vi "new_UI.vi"() -> ()   [LabVIEW 2019]
uses:
  Classes/Assembly/Assembly Run.lvclass
  Classes/Workspace/Fixture Enum.ctl
  Classes/Workspace/Fixture.lvclass
  Classes/Controller/Controller.lvclass
  Classes/Routine/Routine Enum.ctl
  Classes/Routine/Routine.lvclass
panel:
  in  "stop":bool
  in  "Add 2":bool
  in  "Go 2":bool
  in  "Cluster":T1
  in  "Remove":bool
  in  "Stage":i32(listbox)=-1
  in  "Add":bool
  in  "Routine":T2=enum."Dispense on Plate"
  in  "Update":bool
  out "Numeric":dbl
  out "Numeric 2":dbl
  in  "Stop":bool
  in  "Go":bool
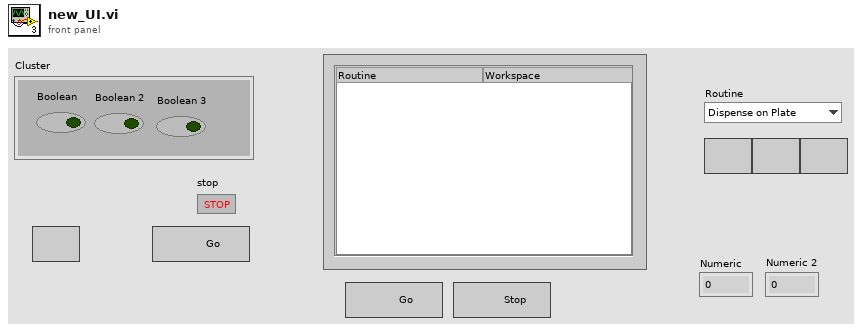
[diagram p1: front panel]
types:
  T1 = cluster{"Boolean":bool, "Boolean 2":bool, "Boolean 3":bool}
  T2 = typedef "Routine.lvclass/Routine Enum.ctl" = enum16{"Primary Pick Up", "Pick Up All", "Put Down Secondary", "Put Down All", "Release Syringe", "Secondary Pick Up", "Secure Syringe", "Dispense on Plate", "Dispense on Kapton", "Dispense on Sensor", "Dispense Offset"}
  T3 = typedef "Fixture.lvclass/Fixture Enum.ctl" = enum16{"Assembly Tray", "Syringe Space", "Component", "Pick Up Tool", "Current Position"}
  T4 = typedef "Controller.lvclass/Controllers.ctl" = cluster{"I-O.lvclass":refnum<class "I-O.lvclass">, "Dispenser.lvclass":refnum<class "Dispenser.lvclass">, "Gantry":refnum<k24>}
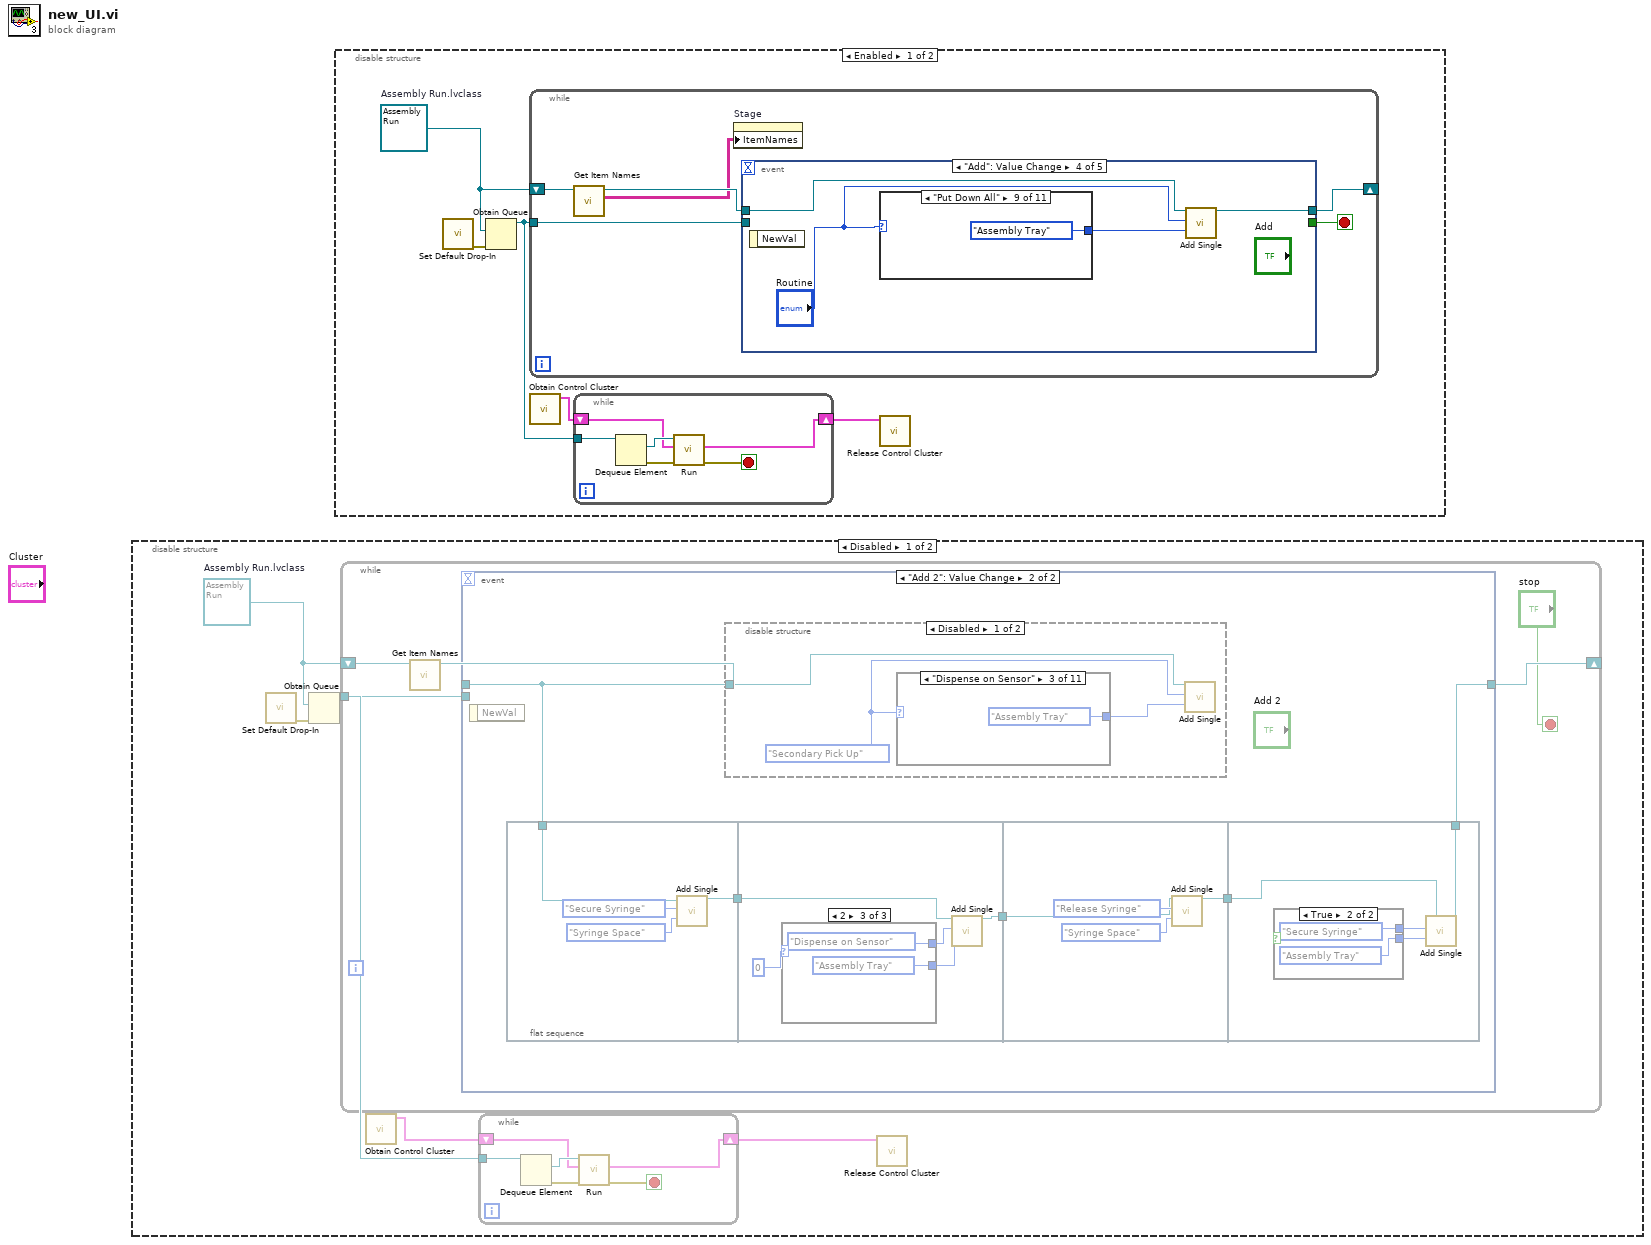
[diagram p0: block diagram]
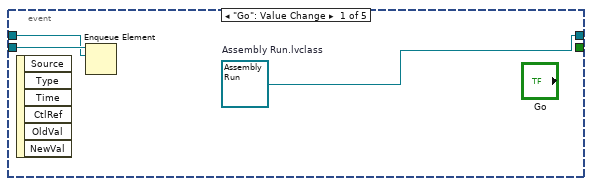
[diagram p2: hidden frame]
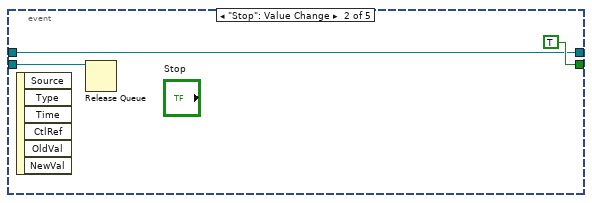
[diagram p3: hidden frame]
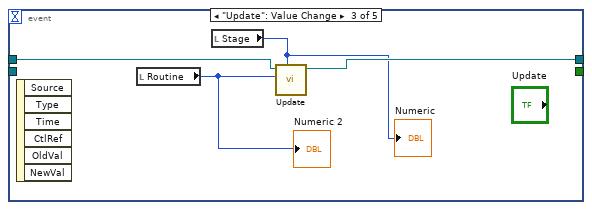
[diagram p4: hidden frame]
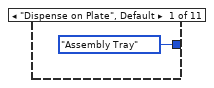
[diagram p5: hidden frame]
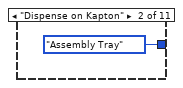
[diagram p6: hidden frame]
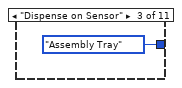
[diagram p7: hidden frame]
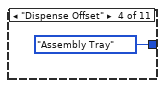
[diagram p8: hidden frame]
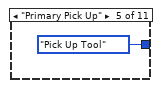
[diagram p9: hidden frame]
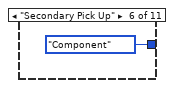
[diagram p10: hidden frame]
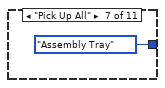
[diagram p11: hidden frame]
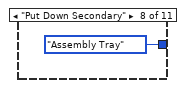
[diagram p12: hidden frame]
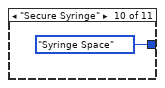
[diagram p13: hidden frame]
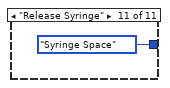
[diagram p14: hidden frame]
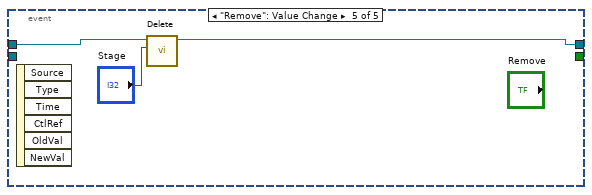
[diagram p15: hidden frame]
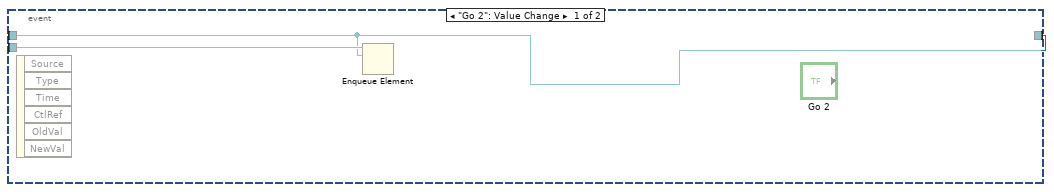
[diagram p17: hidden frame]
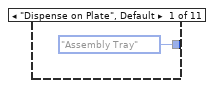
[diagram p18: hidden frame]
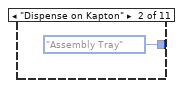
[diagram p19: hidden frame]
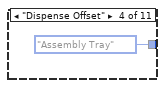
[diagram p20: hidden frame]
diagram:
  n1 = disable-structure shown="Disabled" {
    frame Disabled {
      w2 = refnum<class "Assembly Run.lvclass"> refnum  # Assembly Run.lvclass
      n2 = call "Set Default Drop-In.vi"() -> ("error out"=w3:errorcluster)  [unwired: 11 in]
      n3 = Obtain Queue(element data type=w2, error in (no error)=w3) -> (queue out=w5:refnum<queue>)  [unwired: 3 in, 2 out]
      n4 = while {
        shift-right: [w13] -> _
        shift-left: w2 -> [w15]
        tunnel: w5 -> [w16]
        stop <- "stop" stop-if-true
        n5 = call "Get Item Names.vi"("Assembly Run in"=w15) -> ("Assembly Run out"=w14:refnum<class "Assembly Run.lvclass">)  [unwired: 8 in, 2 out]
        n6 = event shown="[1] \"Add 2\": Value Change" {
          selector: _ -> [_ _]
          dyn-events: _ -> [_ _]
          timeout: _ -> [_ _]
          tunnel: w14 -> [w17 w23]
          tunnel: [w17 w19] -> w13
          tunnel: w16 -> [w18 _]
          event "Go 2": Value Change {
            n7 = event-data() -> ()  [unwired: 1 in, 6 out]
            n8 = Enqueue Element(queue=w18, element=w17) -> ()  [unwired: 2 in, 3 out]
          }
          event "Add 2": Value Change {
            n9 = event-data() -> ()  [unwired: 1 in, 1 out]
            n10 = flat-sequence {
              tunnel: w23 -> [w39]
              tunnel: [w38] -> w22
              tunnel: w22 -> [w44]
              tunnel: [w43] -> w21
              tunnel: w21 -> [w54]
              tunnel: [w53] -> w20
              tunnel: w20 -> [w58]
              tunnel: [w57] -> w19
              frame #0 {
                n11 = call-dynamic "Add Single.vi"("UI in"=w39, "Routine"=Routine_Enum."Secure Syringe" ("Routine 2"), "Fixture"=Fixture_Enum."Syringe Space") -> ("UI out"=w38:refnum<class "Assembly Run.lvclass">)  [unwired: 15 in, 1 out]
              }
              frame #1 {
                n12 = case shown="2" 0 {
                  tunnel: [Fixture_Enum."Assembly Tray" ("Fixture") Fixture_Enum."Assembly Tray" ("Fixture") Fixture_Enum."Assembly Tray" ("Fixture")] -> w46
                  tunnel: [Routine_Enum."Dispense Offset" ("Routine 2") Routine_Enum."Dispense on Plate" ("Routine 2") Routine_Enum."Dispense on Sensor" ("Routine 2")] -> w45
                  frame 0 {
                  }
                  frame 1 {
                  }
                  frame 2 {
                  }
                }
                n13 = call-dynamic "Add Single.vi"("UI in"=w44, "Routine"=w45, "Fixture"=w46) -> ("UI out"=w43:refnum<class "Assembly Run.lvclass">)  [unwired: 15 in, 1 out]
              }
              frame #2 {
                n14 = call-dynamic "Add Single.vi"("UI in"=w54, "Routine"=Routine_Enum."Release Syringe" ("Routine 2"), "Fixture"=Fixture_Enum."Syringe Space") -> ("UI out"=w53:refnum<class "Assembly Run.lvclass">)  [unwired: 15 in, 1 out]
              }
              frame #3 {
                n15 = case shown="True" {
                  selector: _ -> [_ _]
                  tunnel: [_ Fixture_Enum."Assembly Tray" ("Fixture")] -> w60
                  tunnel: [_ Routine_Enum."Secure Syringe" ("Routine 2")] -> w59
                  frame False {
                  }
                  frame True {
                  }
                }
                n16 = call-dynamic "Add Single.vi"("UI in"=w58, "Routine"=w59, "Fixture"=w60) -> ("UI out"=w57:refnum<class "Assembly Run.lvclass">)  [unwired: 15 in, 1 out]
              }
            }
            n17 = disable-structure shown="Disabled" {
              disable-tunnel: w23 -> [w24 _]
              frame Disabled {
                w26 = Routine_Enum."Secondary Pick Up" ("Routine 2")
                n18 = case shown="\"Dispense on Sensor\"" w26 {
                  tunnel: [Fixture_Enum."Assembly Tray" ("Fixture") Fixture_Enum."Assembly Tray" ("Fixture") Fixture_Enum."Assembly Tray" ("Fixture") Fixture_Enum."Assembly Tray" ("Fixture") Fixture_Enum."Pick Up Tool" ("Fixture") Fixture_Enum."Component" ("Fixture") Fixture_Enum."Assembly Tray" ("Fixture") Fixture_Enum."Assembly Tray" ("Fixture") Fixture_Enum."Assembly Tray" ("Fixture") Fixture_Enum."Syringe Space" ("Fixture") Fixture_Enum."Syringe Space" ("Fixture")] -> w25
                  frame "Dispense on Plate", Default {
                  }
                  frame "Dispense on Kapton" {
                  }
                  frame "Dispense on Sensor" {
                  }
                  frame "Dispense Offset" {
                  }
                  frame "Primary Pick Up" {
                  }
                  frame "Secondary Pick Up" {
                  }
                  frame "Pick Up All" {
                  }
                  frame "Put Down Secondary" {
                  }
                  frame "Put Down All" {
                  }
                  frame "Secure Syringe" {
                  }
                  frame "Release Syringe" {
                  }
                }
                n19 = call-dynamic "Add Single.vi"("UI in"=w24, "Routine"=w26, "Fixture"=w25) -> ()  [unwired: 15 in, 2 out]
              }
              frame Enabled {
              }
            }
          }
        }
      }
      n20 = call "Obtain Control Cluster.vi"() -> ("Control Out"=w1:T4)  [unwired: 11 in]
      n21 = while {
        tunnel: w5 -> [w11]
        shift-right: [w6] -> w4
        shift-left: w1 -> [w7]
        stop <- w8 stop-if-true
        n22 = Dequeue Element(queue=w11) -> (element=w10:refnum<class "Assembly Run.lvclass">, error out=w9:errorcluster)  [unwired: 2 in, 2 out]
        n23 = call "Run.vi"("error in (no error)"=w9, "Control In"=w7, "Assembly In"=w10) -> ("error out"=w8:errorcluster, "Control Out"=w6:T4)  [unwired: 6 in, 1 out]
      }
      n24 = call "Release Control Cluster.vi"("output cluster"=w4) -> ()  [unwired: 11 in]
    }
    frame Enabled {
    }
  }
  n25 = disable-structure shown="Enabled" {
    frame Enabled {
      w64 = refnum<class "Assembly Run.lvclass"> refnum  # Assembly Run.lvclass
      n26 = call "Set Default Drop-In.vi"() -> ("error out"=w65:errorcluster)  [unwired: 11 in]
      n27 = Obtain Queue(element data type=w64, error in (no error)=w65) -> (queue out=w67:refnum<queue>)  [unwired: 3 in, 2 out]
      n28 = while {
        shift-right: [w75] -> _
        shift-left: w64 -> [w77]
        tunnel: w67 -> [w78]
        stop <- w79 stop-if-true
        n29 = call "Get Item Names.vi"("Assembly Run in"=w77) -> ("Item names"=w74:string[][], "Assembly Run out"=w76:refnum<class "Assembly Run.lvclass">)  [unwired: 8 in, 1 out]
        n30 = property on="Stage" class="MCListbox (strict)"("ItemNames"=w74) -> ()  [unwired: 2 in, 2 out]
        n31 = event shown="[3] \"Add\": Value Change" {
          selector: _ -> [_ _ _ _ _]
          dyn-events: _ -> [_ _ _ _ _]
          timeout: _ -> [_ _ _ _ _]
          tunnel: [_ TRUE _ _ _] -> w79
          tunnel: w76 -> [w81 w84 w89 w93 w107]
          tunnel: [w80 w84 w88 w92 w106] -> w75
          tunnel: w78 -> [w82 w83 _ _ _]
          event "Go": Value Change {
            w80 = refnum<class "Assembly Run.lvclass"> refnum  # Assembly Run.lvclass
            n32 = event-data() -> ()  [unwired: 1 in, 6 out]
            n33 = Enqueue Element(queue=w82, element=w81) -> ()  [unwired: 2 in, 3 out]
          }
          event "Stop": Value Change {
            n34 = event-data() -> ()  [unwired: 1 in, 6 out]
            n35 = Release Queue(queue=w83) -> ()  [unwired: 2 in, 3 out]
          }
          event "Update": Value Change {
            n36 = event-data() -> ()  [unwired: 1 in, 6 out]
            n37 = local read "Routine"() -> (w86:T2)
            "Numeric 2" <- w86
            n38 = local read "Stage"() -> (w87:i32)
            "Numeric" <- w87
            n39 = call "Update.vi"("Row"=w87, "Routine"=w86, "Assembly Run in"=w89) -> ("Assembly Run out"=w88:refnum<class "Assembly Run.lvclass">)  [unwired: 7 in, 1 out]
          }
          event "Add": Value Change {
            n40 = event-data() -> ()  [unwired: 1 in, 1 out]
            n41 = case shown="\"Put Down All\"" "Routine" {
              tunnel: [Fixture_Enum."Assembly Tray" ("Fixture") Fixture_Enum."Assembly Tray" ("Fixture") Fixture_Enum."Assembly Tray" ("Fixture") Fixture_Enum."Assembly Tray" ("Fixture") Fixture_Enum."Pick Up Tool" ("Fixture") Fixture_Enum."Component" ("Fixture") Fixture_Enum."Assembly Tray" ("Fixture") Fixture_Enum."Assembly Tray" ("Fixture") Fixture_Enum."Assembly Tray" ("Fixture") Fixture_Enum."Syringe Space" ("Fixture") Fixture_Enum."Syringe Space" ("Fixture")] -> w91
              frame "Dispense on Plate", Default {
              }
              frame "Dispense on Kapton" {
              }
              frame "Dispense on Sensor" {
              }
              frame "Dispense Offset" {
              }
              frame "Primary Pick Up" {
              }
              frame "Secondary Pick Up" {
              }
              frame "Pick Up All" {
              }
              frame "Put Down Secondary" {
              }
              frame "Put Down All" {
              }
              frame "Secure Syringe" {
              }
              frame "Release Syringe" {
              }
            }
            n42 = call-dynamic "Add Single.vi"("UI in"=w93, "Routine"="Routine", "Fixture"=w91) -> ("UI out"=w92:refnum<class "Assembly Run.lvclass">)  [unwired: 15 in, 1 out]
          }
          event "Remove": Value Change {
            n43 = event-data() -> ()  [unwired: 1 in, 6 out]
            n44 = call "Delete.vi"("Index"="Stage", "Assembly In"=w107) -> ("Assembly Out"=w106:refnum<class "Assembly Run.lvclass">)  [unwired: 8 in, 1 out]
          }
        }
      }
      n45 = call "Obtain Control Cluster.vi"() -> ("Control Out"=w63:T4)  [unwired: 11 in]
      n46 = while {
        tunnel: w67 -> [w73]
        shift-right: [w68] -> w66
        shift-left: w63 -> [w69]
        stop <- w70 stop-if-true
        n47 = Dequeue Element(queue=w73) -> (element=w72:refnum<class "Assembly Run.lvclass">, error out=w71:errorcluster)  [unwired: 2 in, 2 out]
        n48 = call "Run.vi"("error in (no error)"=w71, "Control In"=w69, "Assembly In"=w72) -> ("error out"=w70:errorcluster, "Control Out"=w68:T4)  [unwired: 6 in, 1 out]
      }
      n49 = call "Release Control Cluster.vi"("output cluster"=w66) -> ()  [unwired: 11 in]
    }
    frame Disabled {
    }
  }
